vi "数据补传对话框.vi"(11 "起始时间":timestamp) -> (0 "参数数值 2":T1, 1 "结束时间输出":timestamp, 2 "起始时间输出":timestamp, 3 "输出":bool=TRUE, 5 "只补小时数据输出":bool)   [LabVIEW 2016, in "数据传输系统-02.lvlib"]
panel:
  in  "只补小时数据":bool
  in  "补传参数":bool
  in  "结束时间":timestamp
  in  "取消":bool
  in  "确定":bool
  # "数据补传时间选择"
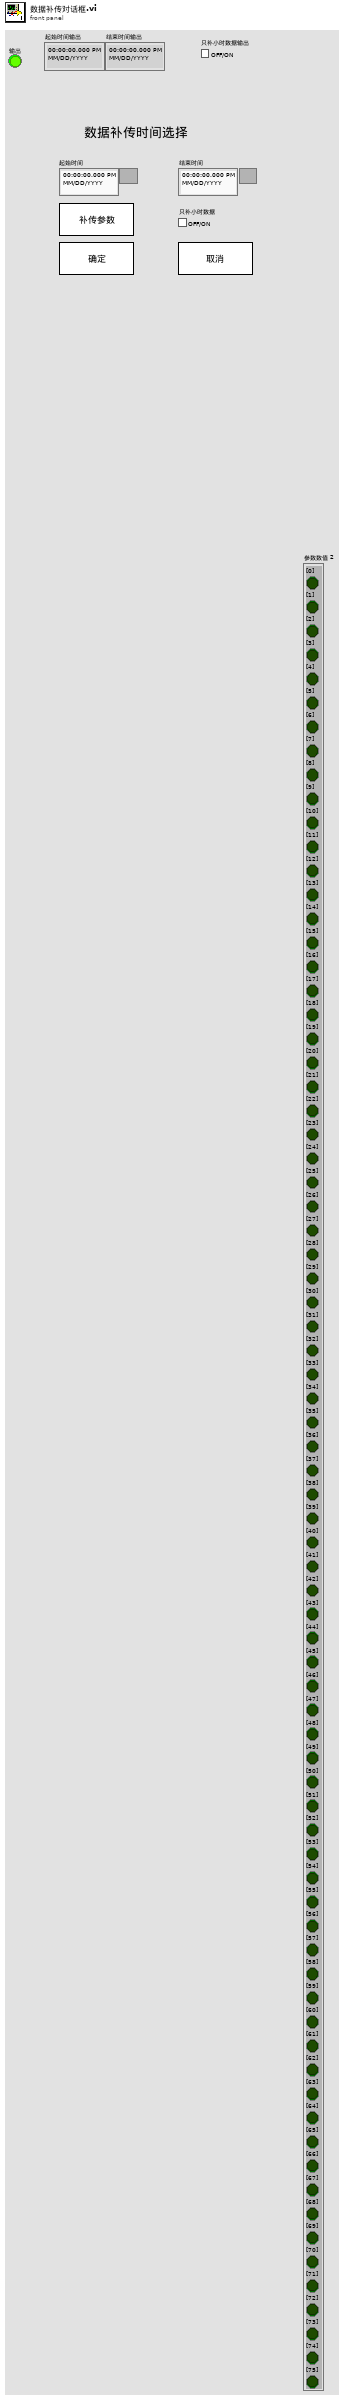
[diagram p1: front panel]
types:
  T1 = cluster{"[0]":bool, "[1]":bool, "[2]":bool, "[3]":bool, "[4]":bool, "[5]":bool, "[6]":bool, "[7]":bool, "[8]":bool, "[9]":bool, "[10]":bool, "[11]":bool, "[12]":bool, "[13]":bool, "[14]":bool, "[15]":bool, "[16]":bool, "[17]":bool, "[18]":bool, "[19]":bool, "[20]":bool, "[21]":bool, "[22]":bool, "[23]":bool, "[24]":bool, "[25]":bool, "[26]":bool, "[27]":bool, "[28]":bool, "[29]":bool, "[30]":bool, "[31]":bool, "[32]":bool, "[33]":bool, "[34]":bool, "[35]":bool, "[36]":bool, "[37]":bool, "[38]":bool, "[39]":bool, "[40]":bool, "[41]":bool, "[42]":bool, "[43]":bool, "[44]":bool, "[45]":bool, "[46]":bool, "[47]":bool, "[48]":bool, "[49]":bool, "[50]":bool, "[51]":bool, "[52]":bool, "[53]":bool, "[54]":bool, "[55]":bool, "[56]":bool, "[57]":bool, "[58]":bool, "[59]":bool, "[60]":bool, "[61]":bool, "[62]":bool, "[63]":bool, "[64]":bool, "[65]":bool, "[66]":bool, "[67]":bool, "[68]":bool, "[69]":bool, "[70]":bool, "[71]":bool, "[72]":bool, "[73]":bool, "[74]":bool, "[75]":bool}
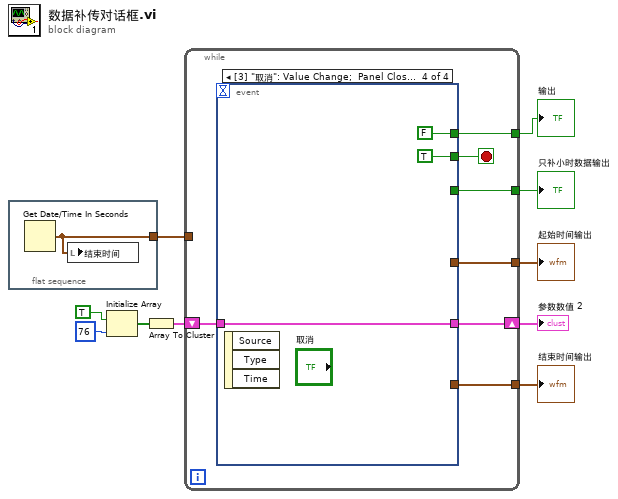
[diagram p0: block diagram]
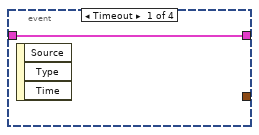
[diagram p2: hidden frame]
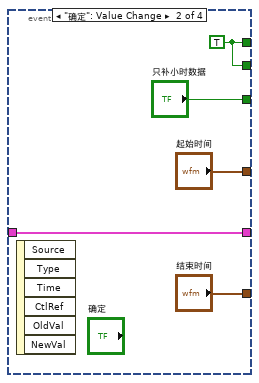
[diagram p3: hidden frame]
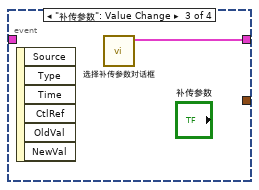
[diagram p4: hidden frame]
diagram:
  n1 = flat-sequence {
    tunnel: [w11] -> w7
    frame #0 {
      n2 = Get Date/Time In Seconds() -> (seconds since 1Jan1904=w11:timestamp)
      n3 = local write "结束时间"(w11) -> ()
    }
  }
  n4 = Initialize Array(TRUE, 76 ("dimension size")) -> (w2:bool[])
  n5 = Array To Cluster(array=w2) -> (cluster=w1:T1)
  n6 = while {
    tunnel: [w18] -> w10
    tunnel: [w16] -> w9
    tunnel: [w15] -> w8
    tunnel: w7 -> [_]
    shift-right: [w14] -> w5
    shift-left: w1 -> [w13]
    tunnel: [w12] -> w6
    stop <- w17 stop-if-true
    n7 = event shown="[3] \"取消\": Value Change;  Panel Close" {
      selector: _ -> [_ _ _ _]
      dyn-events: _ -> [_ _ _ _]
      timeout: _ -> [_ _ _ _]
      tunnel: [_ w24 _ FALSE] -> w18
      tunnel: [_ w24 _ TRUE] -> w17
      tunnel: [_ "起始时间" _ _] -> w16
      tunnel: [_ "结束时间" _ _] -> w15
      tunnel: [w19 w21 w25 w26] -> w14
      tunnel: w13 -> [w19 w21 _ w26]
      tunnel: [_ "只补小时数据" _ _] -> w12
      event Timeout {
        n8 = event-data() -> ()  [unwired: 1 in, 3 out]
      }
      event "确定": Value Change {
        w24 = TRUE
        n9 = event-data() -> ()  [unwired: 1 in, 6 out]
      }
      event "补传参数": Value Change {
        n10 = event-data() -> ()  [unwired: 1 in, 6 out]
        n11 = call "选择补传参数对话框.vi"() -> ("参数数值 2"=w25:T1)  [unwired: 11 in]
      }
      event "取消": Value Change; Panel Close {
        n12 = event-data() -> ()  [unwired: 1 in, 3 out]
      }
    }
  }
  "输出" <- w10
  "起始时间输出" <- w9
  "结束时间输出" <- w8
  "只补小时数据输出" <- w6
  "参数数值 2" <- w5
